vi "Configure Arm Alarm.vi"(4 "RepeatCount":i32 format="%.0g", 5 "Period":dbl, 6 "TimeFraction":dbl, 7 "TimeSeconds":dbl, 8 "error in (no error)":errorcluster {"code" format="%.0x"}, 9 "Enabled (Off)":bool, 10 "AlarmName":string="ALARM0" caption="AlarmName (ALARM0)", 11 "instrument handle":refnum<k15>) -> (0 "error out":errorcluster {"code" format="%.0x"}, 3 "instrument handle out":refnum<k15>)   [LabVIEW 2009, in "Keysight XSAn.lvlib"]
doc: "This VI configures the most commonly configured properties of the arm alarm sub-system.\n\nSupported Models: N9000A, N9000B, N9010A, N9010B, N9020A, N9020B, N9030A, N9030B, N9038A, SPN9003A, SPN9026A"
uses:
  <instrlib>/Keysight XSAn/Keysight XSAn.lvlib
  AgXSAn.dll
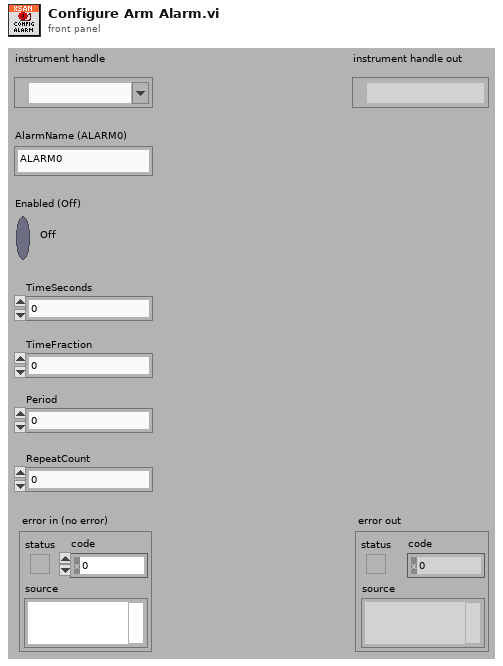
[diagram p1: front panel]
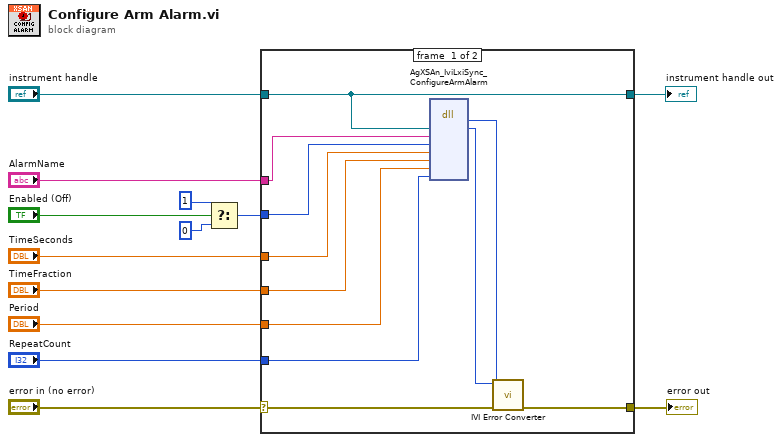
[diagram p0: block diagram]
diagram:
  n1 = Select(t=u16 1, s="Enabled (Off)", f=u16 0) -> (s? t:f=w6:u16)
  n2 = case shown="No Error" "error in (no error)" {
    selector: "error in (no error)" -> [w22 w26]
    tunnel: [w21 w26] -> w13
    tunnel: "instrument handle" -> [w15 w25]
    tunnel: "AlarmName" -> [w20 _]
    tunnel: w6 -> [w19 _]
    tunnel: "TimeSeconds" -> [w14 _]
    tunnel: "TimeFraction" -> [w18 _]
    tunnel: "Period" -> [w17 _]
    tunnel: "RepeatCount" -> [w16 _]
    tunnel: [w15 w25] -> w1
    frame #0 {
      n3 = dll-call lib="AgXSAn**.dll" fn="AgXSAn_IviLxiSync_ConfigureArmAlarm"("Vi"=w15, "AlarmName"=w20, "Enabled"=w19, "TimeSeconds"=w14, "TimeFraction"=w18, "Period"=w17, "RepeatCount"=w16) -> (w23:i32, "Vi"=w24:u32)  [unwired: 9 in, 2 out]
      n4 = call <instrlib>:"IVI Error Converter.vi"("error in (no error)"=w22, "IVI error code (0)"=w23, "instrument handle"=w24) -> ("error out"=w21:errorcluster)  [unwired: 7 in, 1 out]
    }
    frame #1 {
    }
  }
  "error out" <- w13
  "instrument handle out" <- w1
